vi "HVBuncher.Initialize.vi"(0 "i ref in":refnum<vi>, 3 "ms timeout (10000)":i32=10000, 5 "error in (no error)":errorcluster) -> (14 "i ref out":refnum<vi>, 15 "DeviceID":string, 16 "PhysicalNames":string[](array[string]), 17 "LogicalNames":string[](array[string]), 18 "timed out":bool, 19 "error out":errorcluster)   [LabVIEW 2014, in "HVBuncher.lvlib"]
doc: "This vi initializes the used objects and reads the device id."
uses:
  HVBuncher.lvlib
  CSCore/BaseProcess/BaseProcess.lvlib
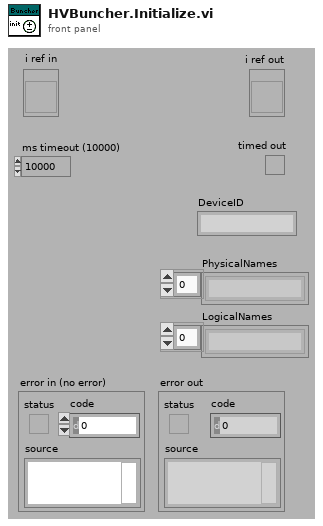
[diagram p1: front panel]
types:
  T1 = typedef "HVBuncher.lvlib/HVBuncher.i attribute.ctl" = cluster{"ObjectsInitialized":bool, "ChildObjects":T2}
  T2 = typedef "HVBuncher.lvlib/HVBuncher.ChildObjects.ctl" = cluster{"ObjectsLoaded":string[], "actVoltage":dbl[]}
  T3 = typedef "BaseProcess.lvlib/BaseProcess.i attribute.ctl" = cluster{"EventStatus":string, "EventError":i32, "PresetEvtWatchD":i32, "PresetPdcWatchD":i32, "EventTimeout":i32, "PeriodicInterval":i32, "Interface":string[], "Address":string[], "Special":string[], "PeriodicError":i32, "PeriodicStatus":string, "SuperProc":string, "Descriptors":T4[], "CaseRef":refnum<vi>, "PdcRef":refnum<vi>, "Thread Ref":refnum<vi>, "eventErrorID":i32, "eventStatusID":i32, "periodicErrorID":i32, "periodicStatusID":i32, "pdcCtrID":i32}
  T4 = typedef "BaseProcess.lvlib/BaseProcess.descriptor definition.ctl" = cluster{"selector":string, "descriptor":T5}
  T5 = typedef "BaseProcess.lvlib/BaseProcess.descriptor string definition.ctl" = string
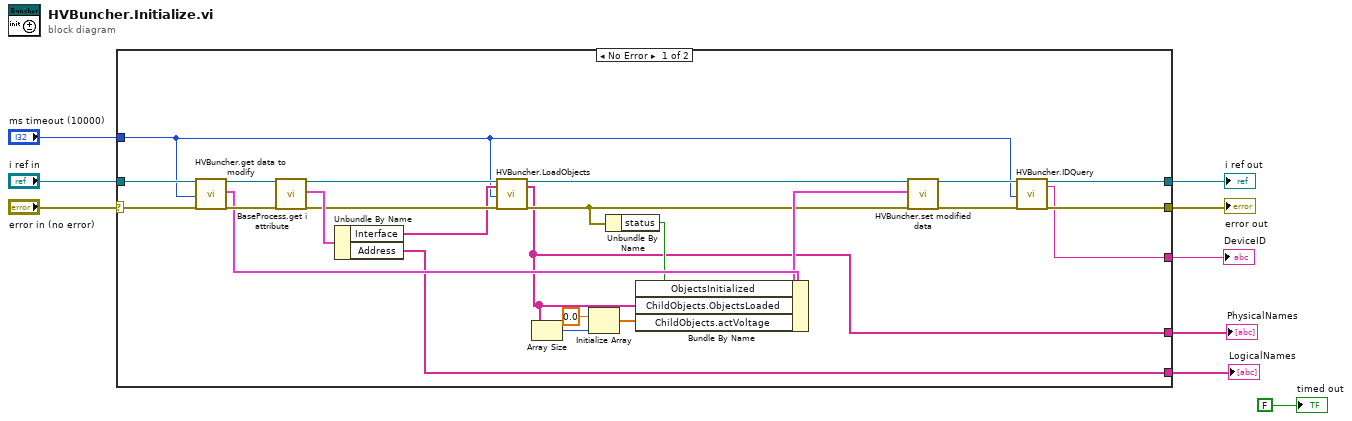
[diagram p0: block diagram]
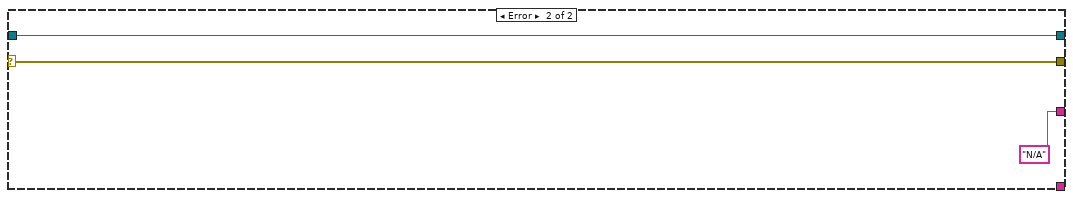
[diagram p2: hidden frame]
diagram:
  n1 = case shown="No Error" "error in (no error)" {
    selector: "error in (no error)" -> [w32 w35]
    tunnel: "i ref in" -> [w33 w36]
    tunnel: [w18 w36] -> w8
    tunnel: [w17 w35] -> w6
    tunnel: "ms timeout (10000)" -> [w15 _]
    tunnel: [w16 "N/A"] -> w3
    tunnel: [w13 _] -> w2
    tunnel: [w14 _] -> w1
    frame No Error {
      n2 = call "HVBuncher.get data to modify.vi"("i ref in"=w33, "ms timeout (10000)"=w15, "error in (no error)"=w32) -> ("i ref out"=w31:refnum<vi>, "i attribute"=w26:T1, "error out"=w30:errorcluster)  [unwired: 13 in, 1 out]
      n3 = call "BaseProcess.get i attribute.vi"("i ref in"=w31, "error in (no error)"=w30) -> ("i ref out"=w28:refnum<vi>, "i attribute"=w29:T3, "error out"=w27:errorcluster)  [unwired: 15 in]
      n4 = Unbundle By Name(w29) -> ("Interface"=w21:string[], "Address"=w14:string[])
      n5 = call "HVBuncher.LoadObjects.vi"("i ref in"=w28, "Objects"=w21, "ms timeout (10000)"=w15, "error in (no error)"=w27) -> ("i ref out"=w25:refnum<vi>, "ObjectsLoaded"=w13:string[], "error out"=w23:errorcluster)  [unwired: 12 in, 1 out]
      n6 = Array Size(array=w13) -> (size(s)=w12:i32)
      n7 = Initialize Array(0.0 ("element"), w12) -> (w11:dbl[])
      n8 = Unbundle By Name(w23) -> ("status"=w22:bool)
      n9 = Bundle By Name(cluster=w26, "ObjectsInitialized"=w22, "ChildObjects.ObjectsLoaded"=w13, "ChildObjects.actVoltage"=w11) -> (w24:T1)
      n10 = call "HVBuncher.set modified data.vi"("i ref in"=w25, "i attribute"=w24, "error in (no error)"=w23) -> ("i ref out"=w20:refnum<vi>, "error out"=w19:errorcluster)  [unwired: 15 in]
      n11 = call "HVBuncher.IDQuery.vi"("i ref in"=w20, "ms timeout (10000)"=w15, "error in (no error)"=w19) -> ("i ref out"=w18:refnum<vi>, "DeviceID"=w16:string, "error out"=w17:errorcluster)  [unwired: 13 in, 1 out]
    }
    frame Error {
    }
  }
  "error out" <- w6
  "i ref out" <- w8
  "DeviceID" <- w3
  "PhysicalNames" <- w2
  "LogicalNames" <- w1
  "timed out" <- FALSE ("timed out")
